vi "RF SandBox.vi"() -> ()   [LabVIEW 2014]
uses:
  <vilib>/NI/Tools/String/Tools_String.lvlib
panel:
  out "Range Finder sensor parsed output":string[](array[string])
  out "?":bool
  out "appended array":string[](array[string])
  in  "Take Point":bool
  in  "stop":bool
  out "x >= y?":bool
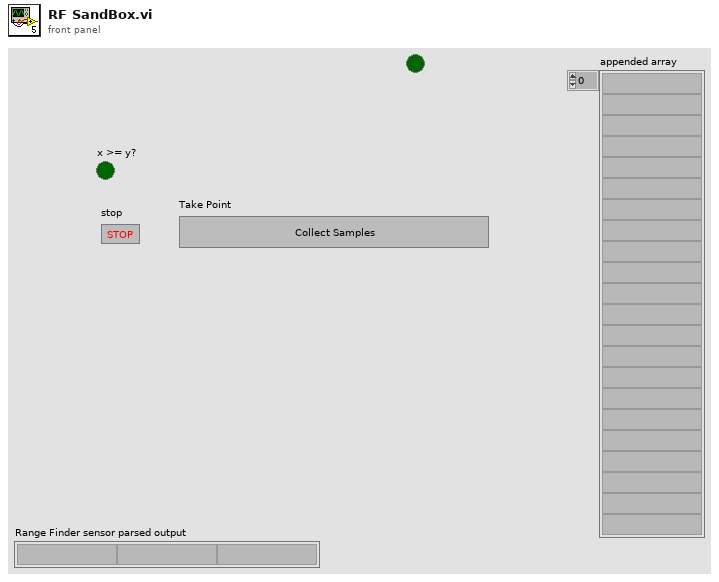
[diagram p1: front panel]
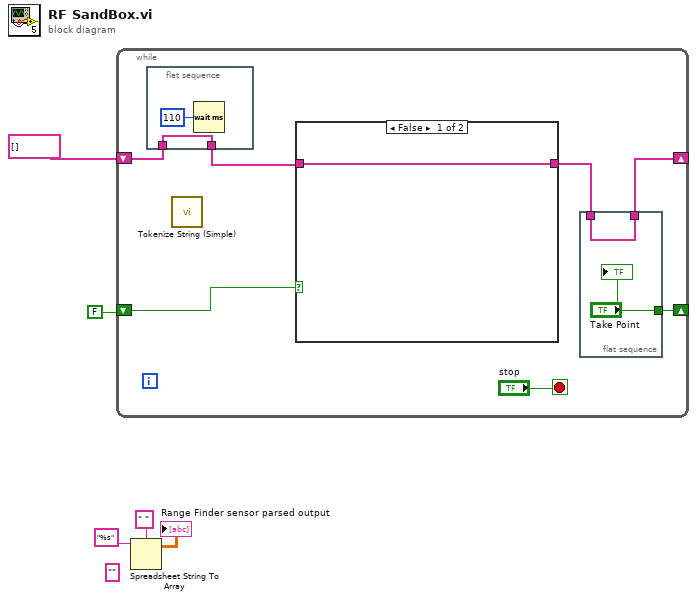
[diagram p0: block diagram]
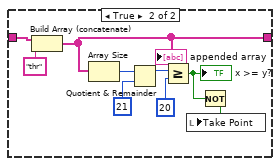
[diagram p2: hidden frame]
diagram:
  (unwired) ""
  n1 = while {
    shift-right: [w7] -> _
    shift-left: string[] [] -> [w10]
    shift-right: [w12] -> _
    shift-left: FALSE -> [w11]
    stop <- "stop" stop-if-true
    n2 = flat-sequence {
      tunnel: w10 -> [w16]
      tunnel: [w16] -> w9
      frame #0 {
        n3 = Wait (ms)(milliseconds to wait=u32 110) -> ()  [unwired: 1 out]
      }
    }
    n4 = call <vilib>:"Tokenize String (Simple).vi"() -> ()  [unwired: 4 in, 2 out]
    n5 = case shown="False" w11 {
      tunnel: w9 -> [w18 w23]
      tunnel: [w18 w21] -> w8
      frame False {
      }
      frame True {
        n6 = Build Array (concatenate)(w23, "thr") -> (w21:string[])
        "appended array" <- w21
        n7 = Array Size(array=w21) -> (size(s)=w24:i32)
        n8 = Quotient & Remainder(x=w24, y=21) -> (x-y*floor(x/y)=w26:i32)  [unwired: 1 out]
        n9 = Greater Or Equal?(x=w26, y=20) -> (x >= y?=w20:bool)
        "x >= y?" <- w20
        n10 = Not(x=w20) -> (.not. x?=w19:bool)
        n11 = local write "Take Point"(w19) -> ()
      }
    }
    n12 = flat-sequence {
      tunnel: ["Take Point"] -> w12
      tunnel: w8 -> [w15]
      tunnel: [w15] -> w7
      frame #0 {
        "?" <- "Take Point"
      }
    }
  }
  n13 = Spreadsheet String To Array(delimiter (Tab)=" ", format string="%s") -> (spreadsheet string=w1:string, array=→"Range Finder sensor parsed output":dbl[][])  [unwired: 1 in]
